vi "Restore Stratup Configuration.vi"(8 "error in (no error)":errorcluster, 10 "Startup Configuration File":path=path "C:/Data/Config/start-up.cfg", 11 "Monitor-Pulse in":refnum<class "Monitor-Pulse.lvclass">) -> (0 "error out":errorcluster, 3 "Monitor-Pulse out":refnum<class "Monitor-Pulse.lvclass">)   [LabVIEW 2015, in "Monitor-Pulse.lvclass"]
uses:
  Monitor-Pulse.lvclass
  Start-up Configuration.ctl
  Module Types.ctl
  Monitor-Pulse.lvclass/Monitor-Pulse.ctl
  <vilib>/Utility/config.llb/NI_LVConfig.lvlib
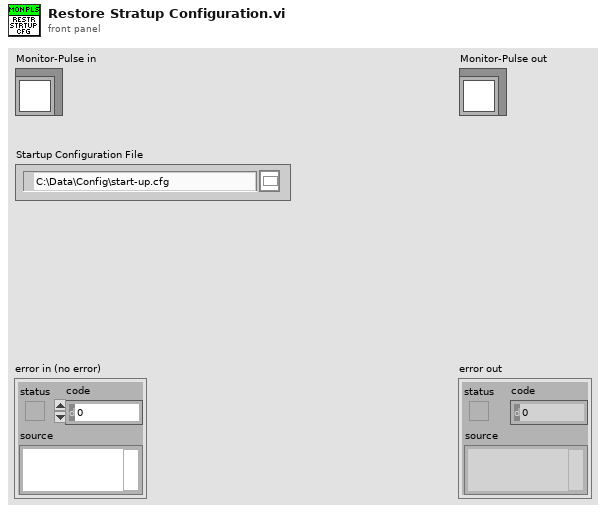
[diagram p1: front panel]
types:
  T1 = typedef "Start-up Configuration.ctl" = cluster{"Load Modules":T2[]}
  T2 = typedef "Module Types.ctl" = enum16{"NONE", "NI-DAQmx", "NI-Scope", "Red Pitaya Digitizer", "GaGe", "VISA Device", "Red Piataya Lockin", "Monitor Controller", "Pulse Controller", "Integrate Pulse"}
  T3 = typedef "NI_LVConfig.lvlib/Config Data RefNum.ctl" = refnum<k1>
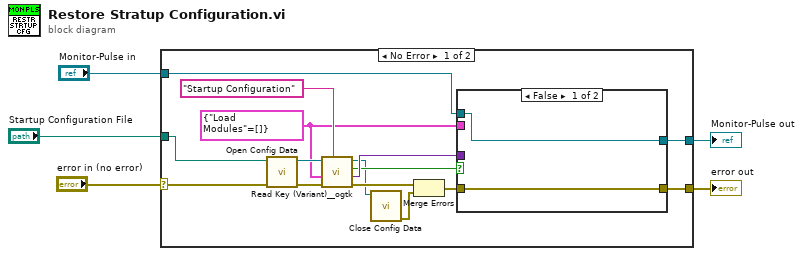
[diagram p0: block diagram]
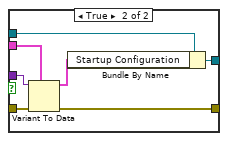
[diagram p2: hidden frame]
diagram:
  n1 = case shown="No Error" "error in (no error)" {
    selector: "error in (no error)" -> [w12 w31]
    tunnel: [w11 w31] -> w4
    tunnel: [w15 w30] -> w2
    tunnel: "Monitor-Pulse in" -> [w20 w30]
    tunnel: "Startup Configuration File" -> [w19 _]
    frame No Error {
      w13 = T1 {"Load Modules"=[]} ("Initial Configuration")
      n2 = call <vilib>:"Open Config Data.vi"("error in (no error)"=w12, "configuration file path"=w19) -> ("error out"=w16:errorcluster, "refnum"=w17:T3)  [unwired: 7 in, 1 out]
      n3 = call <userlib>:"Read Key (Variant)__ogtk.vi"("section"="Startup Configuration", "error in (no error)"=w16, "type"=w13, "refnum"=w17) -> ("error out"=w9:errorcluster, "key-value"=w14:variant, "found?"=w10:bool, "refnum out"=w8:T3)  [unwired: 4 in]
      n4 = call <vilib>:"Close Config Data.vi"("refnum"=w8) -> ("error out"=w7:errorcluster)  [unwired: 9 in, 1 out]
      n5 = Merge Errors(w9, w7) -> (w6:errorcluster)
      n6 = case shown="False" w10 {
        tunnel: w20 -> [w22 w29]
        tunnel: [w22 w28] -> w15
        tunnel: w6 -> [w21 w27]
        tunnel: w14 -> [_ w26]
        tunnel: w13 -> [_ w25]
        tunnel: [w21 w23] -> w11
        frame False {
        }
        frame True {
          n7 = Variant To Data(error in=w27, type=w25, Variant=w26) -> (data=w24:T1, error out=w23:errorcluster)
          n8 = Bundle By Name(cluster=w29, "Startup Configuration"=w24) -> (w28:refnum<class "Monitor-Pulse.lvclass">)
        }
      }
    }
    frame Error {
    }
  }
  "error out" <- w4
  "Monitor-Pulse out" <- w2
